vi "Max Time Cruise.vi"(1 "Angle Displacement":dbl, 2 "Max Acceleration":dbl, 3 "Max Velocity":dbl) -> (0 "Max Time Cruise":dbl)   [LabVIEW 2015]
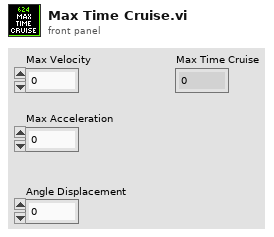
[diagram p1: front panel]
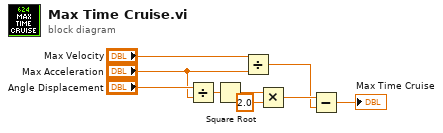
[diagram p0: block diagram]
diagram:
  n1 = Divide(x="Angle Displacement", y="Max Acceleration") -> (x/y=w8:dbl)
  n2 = Square Root(x=w8) -> (sqrt(x)=w7:dbl)
  n3 = Divide(x="Max Velocity", y="Max Acceleration") -> (x/y=w2:dbl)
  n4 = Multiply(x=w7, y=2.0) -> (x*y=w3:dbl)
  n5 = Subtract(x=w3, y=w2) -> (x-y=→"Max Time Cruise":dbl)
